vi "Unravel_ScaniValve.vi"(1 "Port Number":u8=1) -> (0 "Port Number out":u8=1 min=1 max=48 step=1)   [LabVIEW 2011]
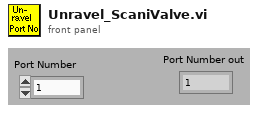
[diagram p1: front panel]
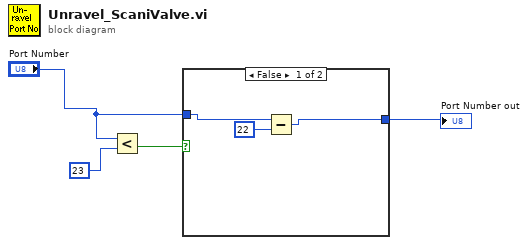
[diagram p0: block diagram]
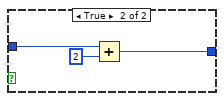
[diagram p2: hidden frame]
diagram:
  n1 = Less?(x="Port Number", y=u8 23) -> (x < y?=w3:bool)
  n2 = case shown="False" w3 {
    tunnel: "Port Number" -> [w7 w10]
    tunnel: [w6 w8] -> w1
    frame False {
      n3 = Subtract(x=w7, y=u8 22) -> (x-y=w6:u8)
    }
    frame True {
      n4 = Add(x=w10, y=u8 2) -> (x+y=w8:u8)
    }
  }
  "Port Number out" <- w1
